vi "Example Threshold.vi"() -> ()   [LabVIEW 2010]
uses:
  C:/tf/play/labview/Tinkerforge.dll
  Tinkerforge.dll
panel:
  out "last z (G)":sgl
  out "last y (G)":sgl
  in  "stop":bool
  out "callback counter":i32
  out "last x (G)":sgl
  in  "uid":string="amb"
  in  "port":i32=4223
  in  "host":string="localhost"
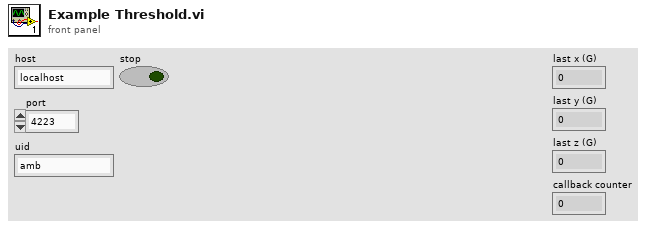
[diagram p1: front panel]
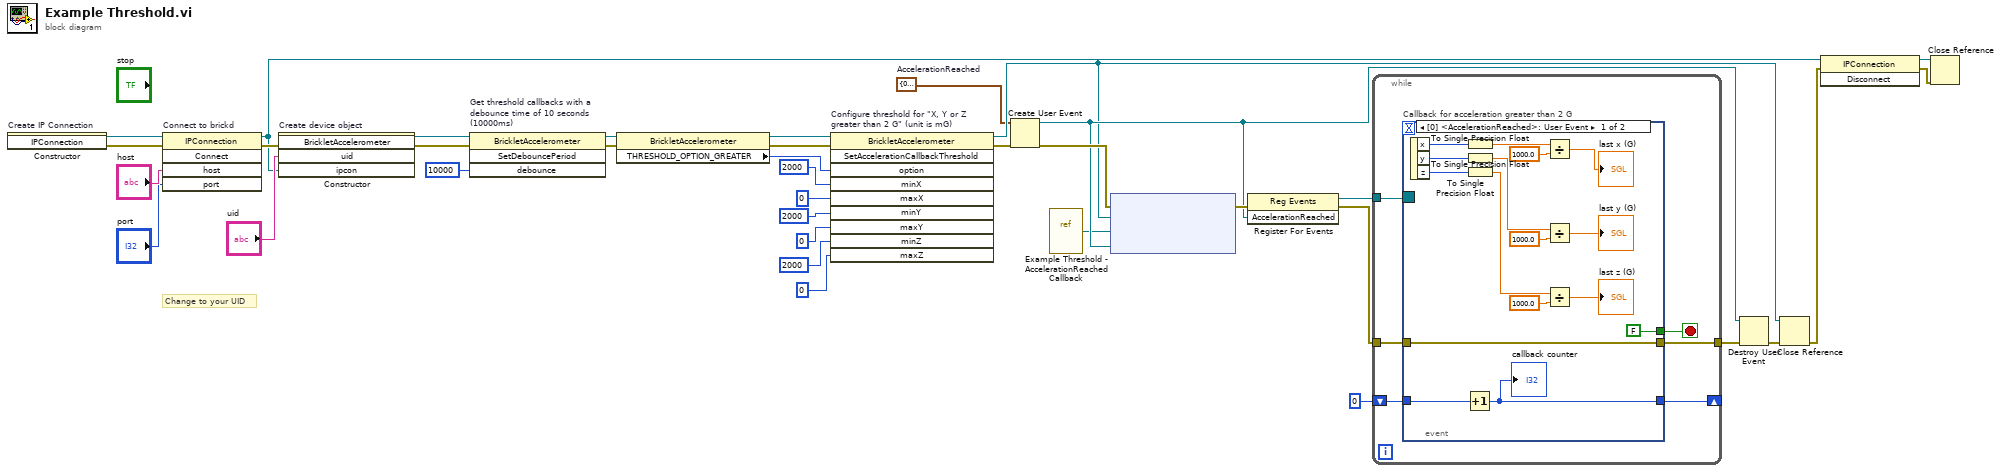
[diagram p0: block diagram]
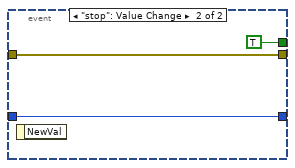
[diagram p2: hidden frame]
diagram:
  w2 = cluster{"x":i16, "y":i16, "z":i16} {"x"=0, "y"=0, "z"=0}  # AccelerationReached
  # "Change to your UID"
  n1 = constructor on="Create IP Connection" class="IPConnection"() -> (reference out=w36:refnum<k24>, error out=w7:errorcluster)  [unwired: 3 in, 1 out]
  n2 = invoke on="Connect to brickd" class="IPConnection" method="Connect"(reference=w36, error in=w7, "host"="host", "port"="port") -> (reference out=w29:refnum<k24>, error out=w32:errorcluster)  [unwired: 1 in, 3 out]
  n3 = constructor on="Create device object" class="BrickletAccelerometer"(error in=w32, "uid"="uid", "ipcon"=w29) -> (reference out=w19:refnum<k24>, error out=w20:errorcluster)  [unwired: 2 in, 3 out]
  n4 = invoke on="Get threshold callbacks with a\ndebounce time of 10 seconds\n(10000ms)" class="BrickletAccelerometer" method="SetDebouncePeriod"(reference=w19, error in=w20, "debounce"=i64 10000 ("period")) -> (reference out=w11:refnum<k24>, error out=w13:errorcluster)  [unwired: 1 in, 2 out]
  n5 = property class="BrickletAccelerometer"(reference=w11, error in=w13) -> (reference out=w10:refnum<k24>, error out=w12:errorcluster, "THRESHOLD_OPTION_GREATER"=w9:u16)
  n6 = invoke on="Configure threshold for \"X, Y or Z\ngreater than 2 G\" (unit is mG)" class="BrickletAccelerometer" method="SetAccelerationCallbackThreshold"(reference=w10, error in=w12, "option"=w9, "minX"=i16 2000 ("min"), "maxX"=i16 0 ("max"), "minY"=i16 2000, "maxY"=i16 0, "minZ"=i16 2000, "maxZ"=i16 0) -> (reference out=w17:refnum<k24>, error out=w16:errorcluster)  [unwired: 1 in, 8 out]
  n7 = Create User Event(user event datatype=w2, error in=w16) -> (user event=w22:refnum<user-event>, error out=w27:errorcluster)
  n8 = vi-ref "Example Threshold - AccelerationReached Callback.vi"() -> ("vi reference"=w1:refnum<vi>)
  n9 = node ("Register Event Callback")(w27, w17, w1, w22) -> (w26:errorcluster)  [unwired: 1 in, 1 out]
  n10 = register-events(error in=w26, w22) -> (reference out=w25:refnum<event-registration>, error out=w23:errorcluster)  [unwired: 1 in]
  n11 = while {
    tunnel: w25 -> [w42]
    tunnel: [w41] -> w24
    tunnel: w23 -> [w40]
    shift-right: [w38] -> _
    shift-left: 0 -> [w39]
    stop <- w37 stop-if-true
    n12 = event "Callback for acceleration greater than 2 G" shown="[0] <AccelerationReached>: User Event" {
      selector: w42 -> [_ _]
      dyn-events: _ -> [_ _]
      timeout: _ -> [_ _]
      tunnel: [w55 w60] -> w41
      tunnel: w40 -> [w55 w60]
      tunnel: w39 -> [w53 w59]
      tunnel: [w52 w59] -> w38
      tunnel: [FALSE TRUE] -> w37
      event User Event {
        n13 = event-data() -> ("x"=w56:i16, "y"=w44:i16, "z"=w43:i16)  [unwired: 1 in]
        n14 = Increment(x=w53) -> (x+1=w52:i32)
        "callback counter" <- w52
        n15 = To Single Precision Float(number=w56) -> (single precision float=w57:sgl)
        n16 = To Single Precision Float(number=w44) -> (single precision float=w49:sgl)
        n17 = To Single Precision Float(number=w43) -> (single precision float=w46:sgl)
        n18 = Divide(x=w57, y=sgl 1000.0) -> (x/y=→"last x (G)":sgl)
        n19 = Divide(x=w49, y=sgl 1000.0) -> (x/y=→"last y (G)":sgl)
        n20 = Divide(x=w46, y=sgl 1000.0) -> (x/y=→"last z (G)":sgl)
      }
      event "stop": Value Change {
        n21 = event-data() -> ()  [unwired: 1 in, 1 out]
      }
    }
  }
  n22 = Destroy User Event(user event=w22, error in=w24) -> (error out=w21:errorcluster)
  n23 = Close Reference(reference=w17, error in (no error)=w21) -> (error out=w31:errorcluster)
  n24 = invoke class="IPConnection" method="Disconnect"(reference=w29, error in=w31) -> (reference out=w28:refnum<k24>, error out=w30:errorcluster)  [unwired: 1 in, 1 out]
  n25 = Close Reference(reference=w28, error in (no error)=w30) -> ()  [unwired: 1 out]
